vi "DB Path.vi"() -> (3 "appended path":path)   [LabVIEW 2020, in "DataBase.lvlib"]
uses:
  DataBase.lvlib
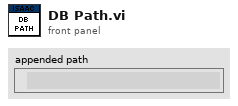
[diagram p1: front panel]
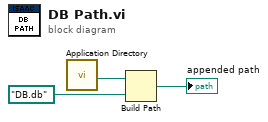
[diagram p0: block diagram]
diagram:
  n1 = call <vilib>:"Application Directory.vi"() -> ("Application Directory"=w3:path)
  n2 = Build Path(base path=w3, name or relative path=path "DB.db") -> (appended path=→"appended path":path)
